vi "CallbackExample - CALLBACK - MouseDownEvent.vi"(4 "User Parameter":T1, 5 "Event Data":T3, 6 "Tree Ref":refnum<vi>, 7 "Event Common Data":cluster{"Source":T4, "Type":T5, "Time":u32} {"Source" items=["LabVIEW UI"=0, "ActiveX"=1, "User Event"=25]}) -> ()   [LabVIEW 2009]
doc: "Demonstration VI that is a callback VI.\n\nAAL 9/09"
uses:
  <vilib>/event_ctls.llb/eventsource.ctl
  <vilib>/event_ctls.llb/lveventtype.ctl
  <vilib>/Utility/miscctls.llb/LVPoint32TypeDef.ctl
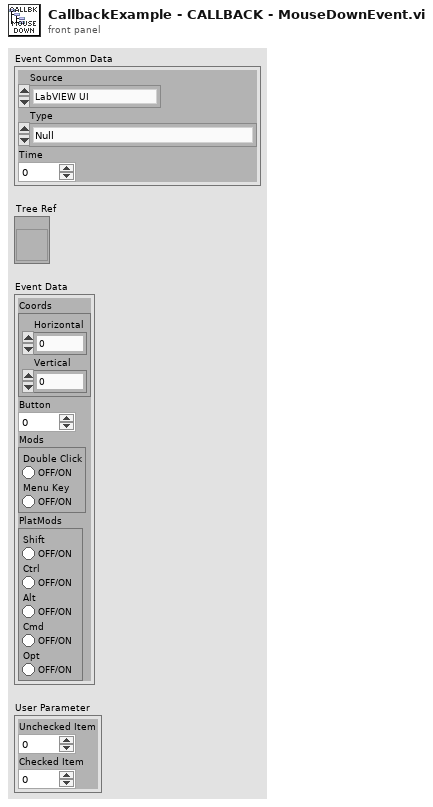
[diagram p1: front panel]
types:
  T1 = cluster{"Unchecked Item":i32, "Checked Item":i32}
  T2 = typedef "LVPoint32TypeDef.ctl" = cluster{"Horizontal":i32, "Vertical":i32}
  T3 = cluster{"Coords":T2, "Button":u16, "Mods":cluster{"Double Click":bool, "Menu Key":bool}, "PlatMods":cluster{"Shift":bool, "Ctrl":bool, "Alt":bool, "Cmd":bool, "Opt":bool}}
  T4 = typedef "eventsource.ctl" = u32
  T5 = typedef "lveventtype.ctl" = enum32{"Null", "Timeout", "App Instance Close", "App Instance Close?", "Cell Edit", "Cell Edit?", "Cursor Grab", "Cursor Grab?", "Cursor Move", "Cursor Release", "Data Change", "Direction Change", "Display State Change", "Drag Ended", "Drag Enter", "Drag Leave", "Drag Over", "Drag Source Update", "Drag Starting", "Drag Starting?", "Drop", "Exec State Change", "Key Down", "Key Down?", "Key Repeat", "Key Repeat?", "Key Up", "Listbox Double Click", "Menu Activation?", "Menu Selection (App)", "Menu Selection? (App)", "Menu Selection (User)", "Mouse Down", "Mouse Down?", "Mouse Enter", "Mouse Leave", "Mouse Move", "Mouse Up", "NI Security User Change (App)", "Pane Size", "Panel Close", "Panel Close?", "Panel Resize", "Plot Attribute Change", "Scale Range Change", "Shortcut Menu Activation?", "Shortcut Menu Selection (App)", "Shortcut Menu Selection? (App)", "Shortcut Menu Selection (User)", "Tree Double Click", "Tree Drag", "Tree Drag?", "Tree Drop", "Tree Drop?", "Tree Item Close", "Tree Item Close?", "Tree Item Open", "Tree Item Open?", "Value Change"}
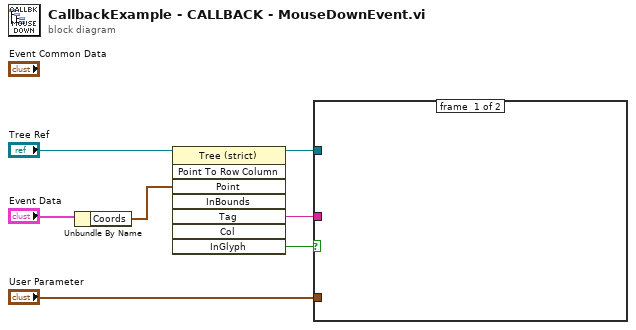
[diagram p0: block diagram]
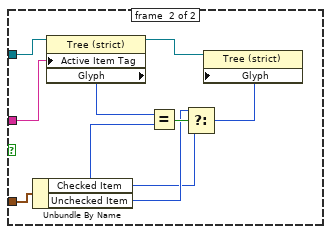
[diagram p2: hidden frame]
diagram:
  n1 = Unbundle By Name("Event Data") -> ("Coords"=w5:T2)
  n2 = invoke class="Tree (strict)" method="Point To Row Column"(reference="Tree Ref", "Point"=w5) -> (reference out=w2:refnum<vi>, "Tag"=w3:string, "InGlyph"=w4:bool)  [unwired: 6 in, 5 out]
  n3 = case shown="True" w4 {
    tunnel: w3 -> [_ w8]
    tunnel: w2 -> [_ w16]
    tunnel: "User Parameter" -> [_ w13]
    frame #0 {
    }
    frame #1 {
      n4 = Unbundle By Name(w13) -> ("Checked Item"=w10:i32, "Unchecked Item"=w11:i32)
      n5 = property class="Tree (strict)"(reference=w16, "Active Item Tag"=w8) -> (reference out=w15:refnum<vi>, "Glyph"=w14:i32)  [unwired: 1 in, 1 out]
      n6 = Equal?(x=w14, y=w10) -> (x = y?=w12:bool)
      n7 = Select(t=w11, s=w12, f=w10) -> (s? t:f=w9:i32)
      n8 = property class="Tree (strict)"(reference=w15, "Glyph"=w9) -> ()  [unwired: 1 in, 2 out]
    }
  }
